vi "LDO Macro Main.vi"() -> ()   [LabVIEW 2020]
uses:
  <vilib>/Utility/file.llb/Read Delimited Spreadsheet (string).vi
panel:
  out "all rows":string[][](array[string])
  in  "Path":path=path "C:/TechnologyLab/NI-2010/Trunk/FVIR and LDO/Macros/Documentation/LDO_test_5_13_2022_9_47_AM.csv"
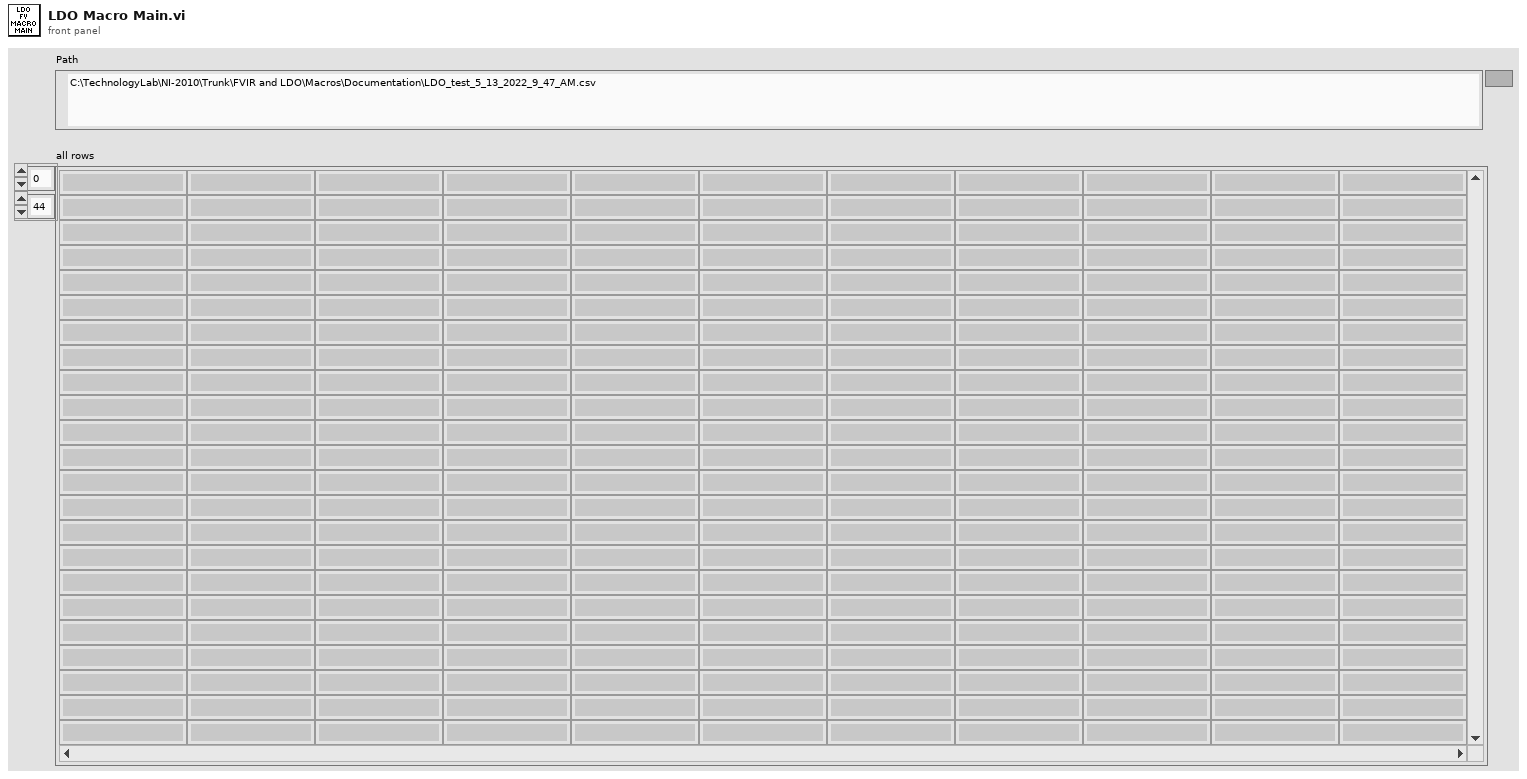
[diagram p1: front panel]
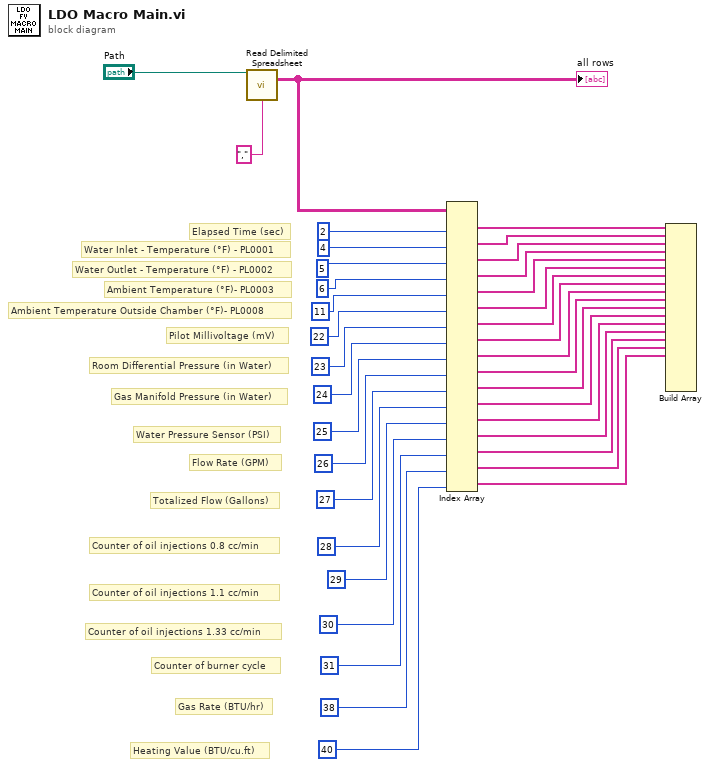
[diagram p0: block diagram]
diagram:
  # "Heating Value (BTU/cu.ft)"
  # "Gas Rate (BTU/hr)"
  # "Counter of burner cycle"
  # "Counter of oil injections 1.33 cc/min"
  # "Counter of oil injections 1.1 cc/min"
  # "Counter of oil injections 0.8 cc/min"
  # "Totalized Flow (Gallons)"
  # "Flow Rate (GPM)"
  # "Water Pressure Sensor (PSI)"
  # "Gas Manifold Pressure (in Water)"
  # "Room Differential Pressure (in Water)"
  # "Pilot Millivoltage (mV)"
  # "Ambient Temperature Outside Chamber (°F)- PL0008"
  # "Ambient Temperature (°F)- PL0003"
  # "Water Outlet - Temperature (°F) - PL0002"
  # "Water Inlet - Temperature (°F) - PL0001"
  # "Elapsed Time (sec)"
  n1 = call-poly <vilib>:"Read Delimited Spreadsheet.vi"("file path (dialog if empty)"="Path", "delimiter (\\t)"="," ("delimiter (\\t)")) -> ("all rows"=w35:string[][])  [unwired: 8 in, 5 out]
  "all rows" <- w35
  n2 = Index Array(array=w35, index (col) #1=2 ("disabled index (col)"), index (col) #2=4 ("index (col)"), index (col) #3=5 ("index (col)"), index (col) #4=6 ("index (col)"), index (col) #5=11 ("index (col)"), index (col) #6=22 ("index (col)"), index (col) #7=23 ("index (col)"), index (col) #8=24 ("index (col)"), index (col) #9=25 ("index (col)"), index (col) #10=26 ("index (col)"), index (col) #11=27 ("index (col)"), index (col) #12=28 ("index (col)"), index (col) #13=29 ("index (col)"), index (col) #14=30 ("index (col)"), index (col) #15=31 ("index (col)"), index (col) #16=38 ("index (col)"), index (col) #17=40 ("index (col)")) -> (element #1=w33:string[], element #2=w30:string[], element #3=w29:string[], element #4=w27:string[], element #5=w25:string[], element #6=w23:string[], element #7=w21:string[], element #8=w19:string[], element #9=w17:string[], element #10=w15:string[], element #11=w13:string[], element #12=w11:string[], element #13=w9:string[], element #14=w7:string[], element #15=w4:string[], element #16=w3:string[], element #17=w1:string[])  [unwired: 17 in]
  n3 = Build Array(w33, w30, w29, w27, w25, w23, w21, w19, w17, w15, w13, w11, w9, w7, w4, w3, w1) -> ()  [unwired: 4 in, 1 out]
